vi "例6-20.vi"() -> ()   [LabVIEW 2019]
uses:
  <vilib>/Analysis/NI_AALPro.lvlib
panel:
  out "残差":dbl format="%.5g"
  out "拟合系数":dbl[](array[numeric]) format="%.6f"
  out "XY图":T1(graph)
  in  "热电势":dbl[](array[numeric]) format="%4_5g"
  in  "输入温度":dbl[](array[numeric])
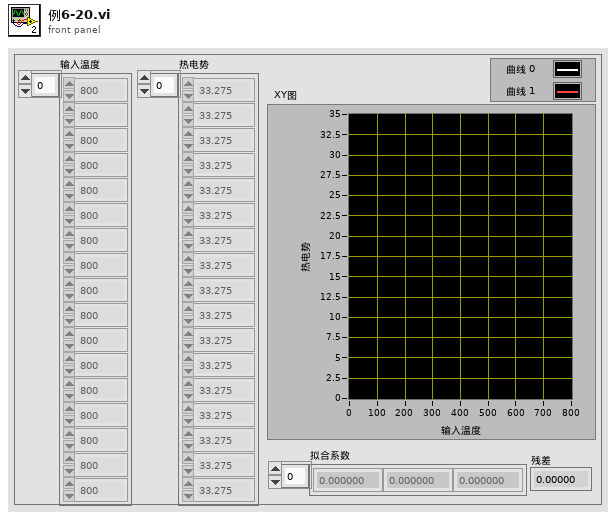
[diagram p1: front panel]
types:
  T1 = cluster{"输入温度":dbl[], "Best Polynomial Fit":dbl[]}[]
  T2 = cluster{"输入温度":dbl[], "Best Polynomial Fit":dbl[]}
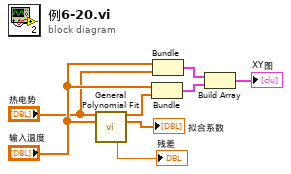
[diagram p0: block diagram]
diagram:
  n1 = call <vilib>:"General Polynomial Fit.vi"("Y"="热电势", "X"="输入温度") -> ("Best Polynomial Fit"=w6:dbl[], "Polynomial Coefficients"=→"拟合系数":dbl[], "residue"=→"残差":dbl)  [unwired: 10 in, 1 out]
  n2 = Bundle("输入温度"="输入温度", "Best Polynomial Fit"=w6) -> (w4:T2)  [unwired: 1 in]
  n3 = Bundle("输入温度"="输入温度", "热电势"="热电势") -> (w5:cluster{"输入温度":dbl[], "热电势":dbl[]})  [unwired: 1 in]
  n4 = Build Array(w5, w4) -> (→"XY图":T1)
